vi "build.event.map.vi"(8 "error in (no error)":errorcluster, 10 "event map in":map{string, set{string}}(c390), 11 "series_class in":refnum<class "series_class.lvclass">) -> (0 "error out":errorcluster, 2 "event map out":map{string, set{string}}(c390), 3 "series_class out":refnum<class "series_class.lvclass">)   [LabVIEW 2024, in "series_class.lvclass"]
uses:
  series_class.lvclass
  series_class.lvclass/series_class.ctl
  issue_class/issue_class.lvclass
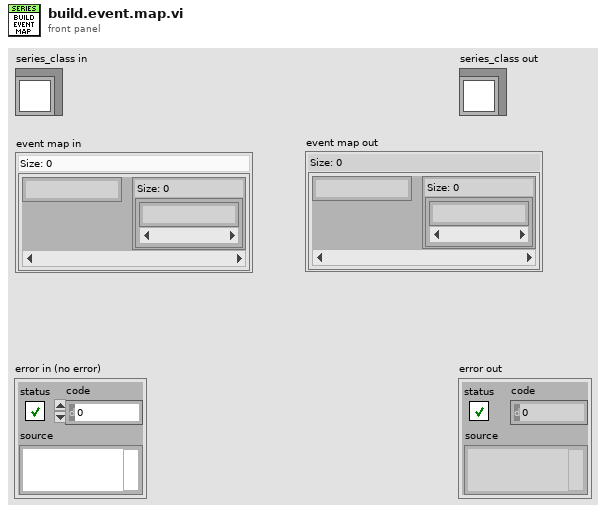
[diagram p1: front panel]
types:
  T1 = typedef "storyArc.ctl" = cluster{"name":string, "url":string}
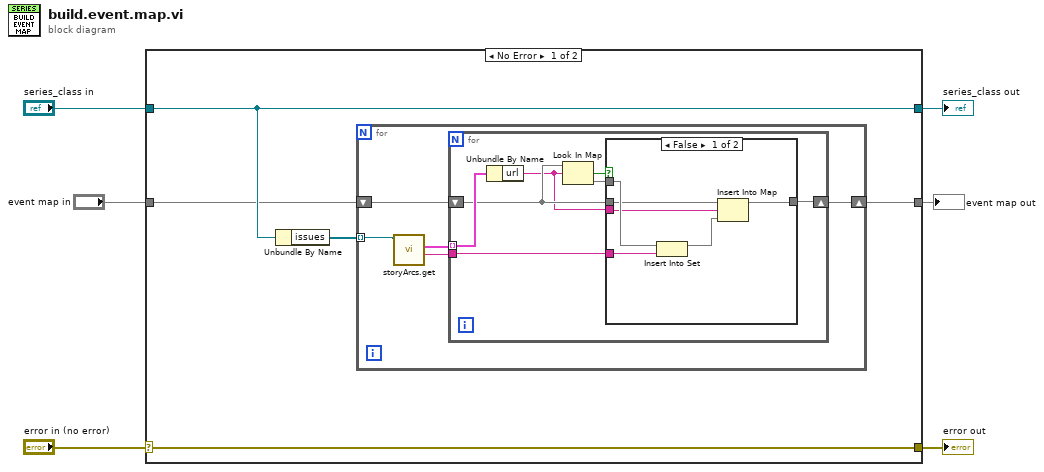
[diagram p0: block diagram]
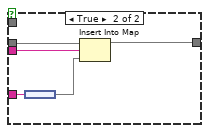
[diagram p2: hidden frame]
diagram:
  n1 = case shown="No Error" "error in (no error)" {
    selector: "error in (no error)" -> [w11 w36]
    tunnel: [w11 w36] -> w5
    tunnel: [w10 w35] -> w3
    tunnel: "series_class in" -> [w10 w35]
    tunnel: "event map in" -> [w8 _]
    tunnel: [w7 _] -> w1
    frame No Error {
      n2 = Unbundle By Name(w10) -> ("issues"=w9:refnum<class "issue_class.lvclass">[])
      n3 = for {
        tunnel: w9 -> [w14] mode=indexing
        shift-right: [w15] -> w7
        shift-left: w8 -> [w16]
        n4 = call "storyArcs.get.vi"("issue_class in"=w14) -> ("id"=w12:string, "storyArcs"=w13:T1[])  [unwired: 7 in, 2 out]
        n5 = for {
          tunnel: w13 -> [w23] mode=indexing
          shift-right: [w18] -> w15
          shift-left: w16 -> [w21]
          tunnel: w12 -> [w19]
          n6 = Unbundle By Name(w23) -> ("url"=w20:string)
          n7 = Look In Map(map=w21, key=w20) -> (key not found?=w22:bool, value=w17:set{string})  [unwired: 1 in]
          n8 = case shown="False" w22 {
            tunnel: w21 -> [w27 w34]
            tunnel: w20 -> [w26 w33]
            tunnel: w19 -> [w28 w32]
            tunnel: [w24 w30] -> w18
            tunnel: w17 -> [w29 _]
            frame False {
              n9 = Insert Into Set(10:w28, 11:w29) -> (3:w25:set{string})  [unwired: 1 out]
              n10 = Insert Into Map(map in=w27, key=w26, value=w25) -> (map out=w24:map{string, set{string}})  [unwired: 2 out]
            }
            frame True {
              n11 = node(w32) -> (w31:set{string})
              n12 = Insert Into Map(map in=w34, key=w33, value=w31) -> (map out=w30:map{string, set{string}})  [unwired: 2 out]
            }
          }
        }
      }
    }
    frame Error {
    }
  }
  "error out" <- w5
  "series_class out" <- w3
  "event map out" <- w1
